vi "Get camera parameter.vi"(8 "error in (no error)":errorcluster, 11 "Cascade512IIBase in":refnum<class "DAQCascade512II.lvclass">) -> (0 "error out":errorcluster, 2 "camera parameters":variant[](array[variant]), 3 "Cascade512IIBase out":refnum<class "DAQCascade512II.lvclass">)   [LabVIEW 2012, in "DAQCascade512II.lvclass"]
uses:
  DAQCascade512II.lvclass
  DAQCascade512II.lvclass/DAQCascade512II.ctl
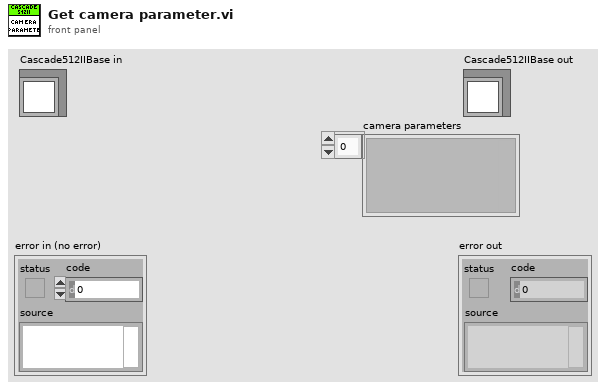
[diagram p1: front panel]
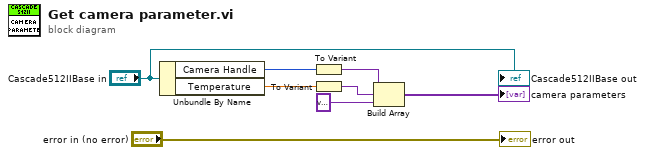
[diagram p0: block diagram]
diagram:
  n1 = Unbundle By Name("Cascade512IIBase in") -> ("Camera Handle"=w6:u32, "Temperature"=w7:dbl)
  n2 = To Variant(anything=w6) -> (Variant=w5:variant)
  n3 = To Variant(anything=w7) -> (Variant=w4:variant)
  n4 = Build Array(w5, w4, variant ("element")) -> (→"camera parameters":variant[])
  "Cascade512IIBase out" <- "Cascade512IIBase in"
  "error out" <- "error in (no error)"
